vi "stopHWEvent.vi"(8 "error in (no error)":errorcluster, 11 "ExperimentControl in":refnum<class "ExperimentControl.lvclass">) -> (0 "error out":errorcluster, 3 "ExperimentControl out":refnum<class "ExperimentControl.lvclass">)   [LabVIEW 2011, in "Views.lvlib" / "ExperimentControl.lvlib" / "ExperimentControl.lvclass"]
uses:
  ExperimentControl.lvclass
  ExperimentControl.lvclass/ExperimentControl.ctl
  Hal/HWController/HWControllerEvents/HWControllerEvents.lvclass
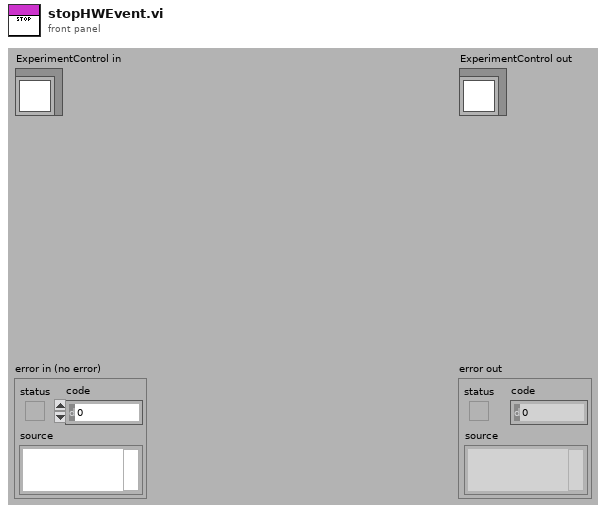
[diagram p1: front panel]
types:
  T1 = enum16{"start", "stop", "statusInquiry", "configure", "resetError", "resourcesInquiry", "reserveResources", "initialise", "resetAllChannels", "staticUpdate", "close", "HWStatus", "error", "resourcesAvailable", "resourcesReserved", "compilerError", "compiledScript", "compilingScript", "runScript", "configureCompiledScript"}
  T2 = enum16{"Ready", "Compiling", "Configured", "Running", "Stopping", "Unresolved Error"}
  T3 = cluster{"incomingEventTypes":cluster{"start":cluster{"Boolean":bool}, "stop":cluster{"Boolean":bool}, "statusInquiry":cluster{"Boolean":bool}, "configure":cluster{"DPScriptPath":path, "TimeStamp":string, "HWLoop?":bool}, "resetError":cluster{"Boolean":bool}, "resourcesInquiry":cluster{"Boolean":bool}, "reserveResources":cluster{"HWList":string[]}, "initialise":cluster{"HWList":string[]}, "close":cluster{"Boolean":bool}, "resetAllChannels":cluster{"Boolean":bool}, "staticChannelUpdate":cluster{"channel_address":string, "calibratedValue":dbl}, "runScript":cluster{"DPScriptPath":path, "TimeStamp":string, "HWLoop?":bool}, "compilingScript":cluster{"Path":path}, "compiledScript":cluster{"Path":path, "timeCompileAt":string}, "compilerError":cluster{"Path":path}, "configureCompiledScript":cluster{"DPScriptPath":path, "TimeStamp":string, "HWLoop?":bool, "CompiledScript":cluster{"ScriptListCompiler.lvclass":refnum<class "ScriptListCompiler.lvclass">, "aoChannels":refnum<class "AnalogOutput.lvclass">[], "doChannels":refnum<class "DigitalOutput.lvclass">[], "rfChannels":refnum<class "DDSOutput.lvclass">[]}}, "restartCompiler":cluster{"restart":bool}, "staticRfChannelUpdate":cluster{"channel_address":string, "Output":cluster{"Frequency(MHz)":dbl, "Amplitude":dbl, "Phase":dbl, "OutputForm":enum16{"Sine", "Square", "Triangle", "Arbitrary"}}}, "cameraUpdate":cluster{"Camera":string, "Type":string, "settings":path}}, "outgoingEventTypes":cluster{"HWStatus":cluster{"status":enum16{"Ready", "Compiling", "Configured", "Running", "Stopping", "Unresolved Error"}}, "error":cluster{"error out":errorcluster}, "resourcesAvailable":cluster{"availableHWList":string[], "reservedHWList":string[]}, "resourcesReserved":cluster{"reservedHWList":string[]}}}
  T4 = cluster{"eventId":enum16{"start", "stop", "statusInquiry", "configure", "resetError", "resourcesInquiry", "reserveResources", "initialise", "resetAllChannels", "staticUpdate", "close", "HWStatus", "error", "resourcesAvailable", "resourcesReserved", "compilerError", "compiledScript", "compilingScript", "runScript", "configureCompiledScript"}, "stop":cluster{"Boolean":bool}}
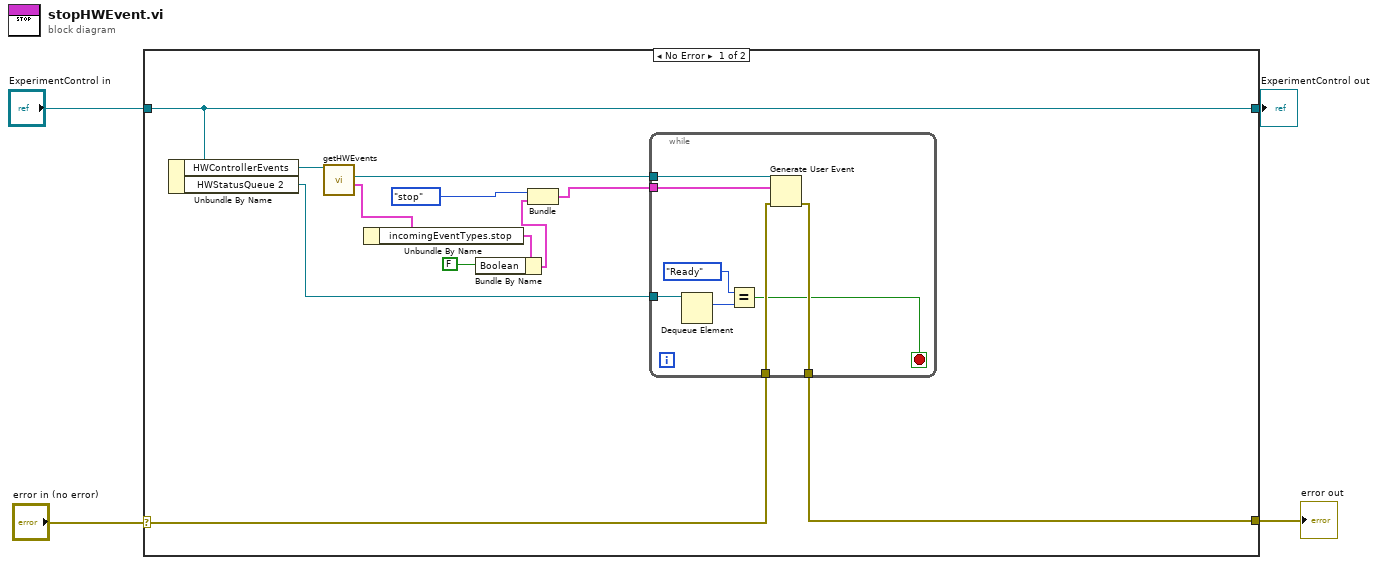
[diagram p0: block diagram]
diagram:
  n1 = case shown="No Error" "error in (no error)" {
    selector: "error in (no error)" -> [w6 w26]
    tunnel: [w7 w26] -> w1
    tunnel: [w16 w25] -> w2
    tunnel: "ExperimentControl in" -> [w16 w25]
    frame No Error {
      n2 = Unbundle By Name(w16) -> ("HWControllerEvents"=w15:refnum<class "HWControllerEvents.lvclass">, "HWStatusQueue 2"=w5:refnum<queue>)
      n3 = call-dynamic "getHWEvents.vi"("HWControllerEvents in"=w15) -> ("eventDataTypes"=w8:T3, "HWCEvent"=w9:refnum<user-event>)  [unwired: 7 in, 2 out]
      n4 = Unbundle By Name(w8) -> ("incomingEventTypes.stop"=w13:cluster{"Boolean":bool})
      n5 = Bundle By Name(cluster=w13, "Boolean"=FALSE) -> (w12:cluster{"Boolean":bool})
      n6 = Bundle("eventId"=T1."stop", "stop"=w12) -> (w14:T4)  [unwired: 1 in]
      n7 = while {
        tunnel: w14 -> [w24]
        tunnel: w9 -> [w23]
        tunnel: [w22] -> w7
        tunnel: w6 -> [w21]
        tunnel: w5 -> [w20]
        stop <- w17 stop-if-true
        n8 = Dequeue Element(queue=w20) -> (element=w18:T2)  [unwired: 2 in, 3 out]
        n9 = Equal?(x=T2."Ready" ("element"), y=w18) -> (x = y?=w17:bool)
        n10 = Generate User Event(user event=w23, event data cluster=w24, error in=w21) -> (error out=w22:errorcluster)  [unwired: 1 out]
      }
    }
    frame Error {
    }
  }
  "error out" <- w1
  "ExperimentControl out" <- w2
